vi "Lab 9 Exercise 6 - Multiplot Graph.vi"() -> ()   [LabVIEW 2023]
panel:
  in  "Square Wave\nFrequecy (Hz)":dbl(slide) scale=0.0..10.0
  in  "Sine Wave\nFrequency (Hz)":dbl(slide) scale=0.0..10.0
  in  "?":bool
  out "Waveform Graph":dynamicdata(graph)
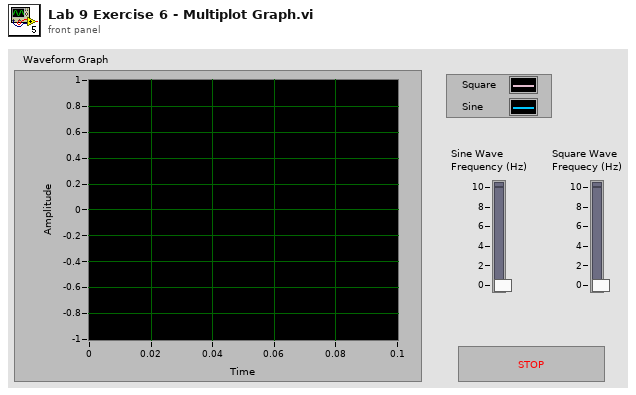
[diagram p1: front panel]
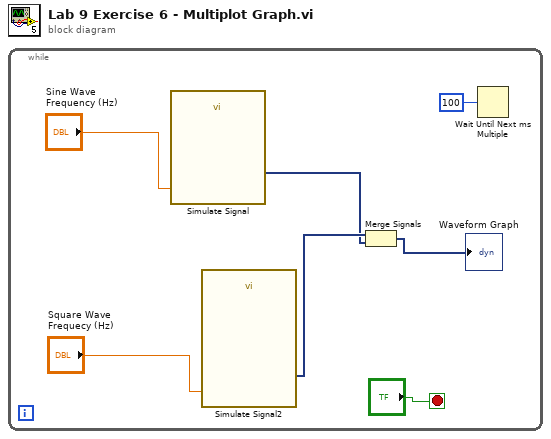
[diagram p0: block diagram]
diagram:
  n1 = while {
    stop <- "?" stop-if-true
    n2 = call "Simulate Signal"("Frequency"="Sine Wave\nFrequency (Hz)") -> ("Sine"=w1:dynamicdata)  [unwired: 13 in, 1 out]
    n3 = call "Simulate Signal2"("Frequency"="Square Wave\nFrequecy (Hz)") -> ("Square"=w3:dynamicdata)  [unwired: 13 in, 1 out]
    n4 = Merge Signals(w3, w1) -> (→"Waveform Graph":dynamicdata)
    n5 = Wait Until Next ms Multiple(millisecond multiple=100) -> ()  [unwired: 1 out]
  }
